vi "Load_Iris.vi"(8 "error in":errorcluster caption="entrée d'erreur") -> (0 "error out":errorcluster caption="sortie d'erreur", 3 "Tableau":string[][](array[string]))   [LabVIEW 2020]
doc: "Data Set Characteristics :\n\nNumber of Instances : 150 (50 in each of three classes)\n\nNumber of Attributes : 4 numeric, predictive attributes and the class\n\nAttribute Information: \n - sepal length in cm\n - sepal width in cm\n - petal length in cm\n - petal width in cm\n\nclass:\n - Iris-Setosa\n - Iris-Versicolour\n - Iris-Virginica\n\nSummary Statistics :\n\nsepal length : 4.3 7.9 5.84 0.83 0.7826\n\nsepal width : 2.0 4.4 3.05 0.43 -0.4194\n\npetal length : 1.0 6.9 3.76 1.76 0.9490 (high!)\n\npetal width : 0.1 2.5 1.20 0.76 0.9565 (high!)\n\nMissing Attribute Values : None\n\nClass Distribution : 33.3% for each of 3 classes.\n\nCreator : R.A. Fisher\n\nDonor : Michael Marshall (MARSHALL%PLU@io.arc.nasa.gov)\n\nDate : July, 1988\n\n\n\n\n\nThe famous Iris database, first used by Sir R.A. Fisher. The dataset is taken from Fisher’s paper. Note that it’s the same as in R, but not as in the UCI Machine Learning Repository, which has two wrong data points.\n\nThis is perhaps the best known database to be found in the pattern recognition literature. Fisher’s paper is a classic in the field and is referenced frequently to this day. (See Duda & Hart, for example.) The data set contains 3 classes of 50 instances each, where each class refers to a type of iris plant. One class is linearly separable from the other 2; the latter are NOT linearly separable from each other."
uses:
  Load_Iris.lvclass
panel:
  out "Load_Iris en sortie":refnum<class "Load_Iris.lvclass">
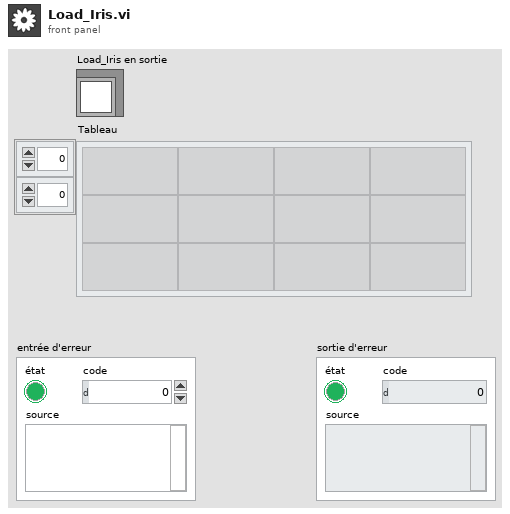
[diagram p1: front panel]
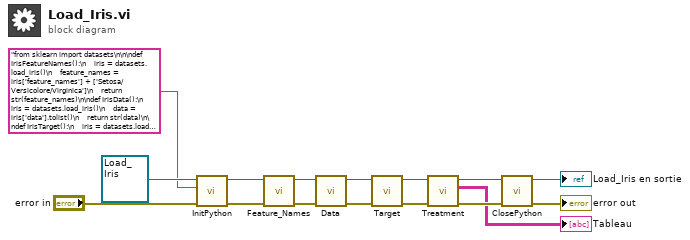
[diagram p0: block diagram]
diagram:
  n1 = call-dynamic "InitPython.vi"("error in (no error)"="error in", "Python Instruction"="from sklearn import datasets\n\n\ndef IrisFeatureNames():\n    iris = datasets.load_iris()\n    feature_names = iris['feature_names'] + ['Setosa/Versicolore/Virginica']\n    return str(feature_names)\n\ndef IrisData():\n    iris = datasets.load_iris()\n    data = iris['data'].tolist()\n    return str(data)\n\ndef IrisTarget():\n    iris = datasets.load_iris()\n    data_target = iris['target'].tolist()\n    return str(data_target)", "Scikit-learn en entrée"=refnum<class "Load_Iris.lvclass"> refnum ("Load_Iris.lvclass")) -> ("error out"=w11:errorcluster, "Scikit-learn en sortie"=w12:refnum<class "Load_Iris.lvclass">)  [unwired: 7 in]
  n2 = call-dynamic "Feature_Names.vi"("error in (no error)"=w11, "Load_Iris en entrée"=w12) -> ("error out"=w9:errorcluster, "Load_Iris en sortie"=w10:refnum<class "Load_Iris.lvclass">)  [unwired: 8 in]
  n3 = call-dynamic "Data.vi"("error in (no error)"=w9, "Load_Iris en entrée"=w10) -> ("error out"=w7:errorcluster, "Load_Iris en sortie"=w8:refnum<class "Load_Iris.lvclass">)  [unwired: 8 in]
  n4 = call-dynamic "Target.vi"("error in (no error)"=w7, "Load_Iris en entrée"=w8) -> ("error out"=w5:errorcluster, "Load_Iris en sortie"=w6:refnum<class "Load_Iris.lvclass">)  [unwired: 8 in]
  n5 = call-dynamic "Treatment.vi"("error in (no error)"=w5, "Load_Iris en entrée"=w6) -> ("error out"=w3:errorcluster, "Tableau"=→"Tableau":string[][], "Load_Iris en sortie"=w4:refnum<class "Load_Iris.lvclass">)  [unwired: 7 in]
  n6 = call-dynamic "ClosePython.vi"("error in (no error)"=w3, "Scikit-learn en entrée"=w4) -> ("error out"=→"error out":errorcluster, "Scikit-learn en sortie"=→"Load_Iris en sortie":refnum<class "Load_Iris.lvclass">)  [unwired: 8 in]
